vi "Cal BC (Numeric).vi"(8 "error in (no error)":errorcluster, 10 "BC in":variant, 11 "Domain_Steady_2D_Rect in":refnum<class "NI_Domain_Steady_2D_Rect.lvclass">) -> (0 "error out":errorcluster, 2 "BC out":variant, 3 "Domain_Steady_2D_Rect out":refnum<class "NI_Domain_Steady_2D_Rect.lvclass">)   [LabVIEW 2017, in "NI_PDE.lvlib" / "NI_Domain_Steady_2D_Rect.lvclass"]
uses:
  <vilib>/gmath/pde.llb/DomainClass/Domain_Steady_2D_Rect/NI_Domain_Steady_2D_Rect.lvclass
  <vilib>/gmath/pde.llb/BCClass/BC_Steady_2D_Numeric/BC Data.ctl
  <vilib>/gmath/pde.llb/Common/PDE_BC Type.ctl
  <vilib>/gmath/pde.llb/Common/PDE_BC Position 2D.ctl
  <vilib>/gmath/pde.llb/DomainClass/Domain_Steady_2D_Rect/NI_Domain_Steady_2D_Rect.lvclass/NI_Domain_Steady_2D_Rect.ctl
  <vilib>/gmath/NI_PDE.lvlib
  <vilib>/gmath/pde.llb/BCClass/BC_Steady_2D_Numeric/NI_BC_Steady_2D_Numeric.lvclass
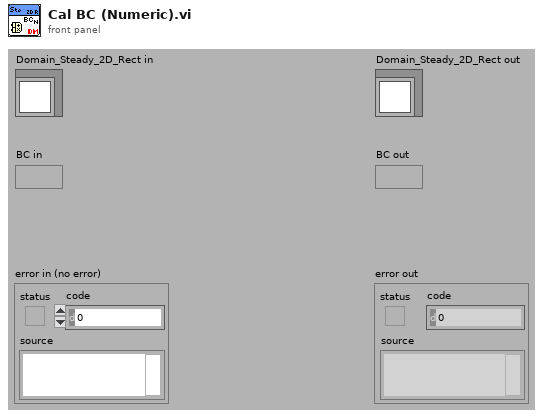
[diagram p1: front panel]
types:
  T1 = typedef "NI_PDE.lvlib/NI_BC_Steady_2D_Numeric.lvclass/BC Data.ctl" = cluster{"type":T2, "position":T3, "G":dbl[]}
  T2 = typedef "NI_PDE.lvlib/PDE_BC Type.ctl" = i32
  T3 = typedef "NI_PDE.lvlib/PDE_BC Position 2D.ctl" = i32
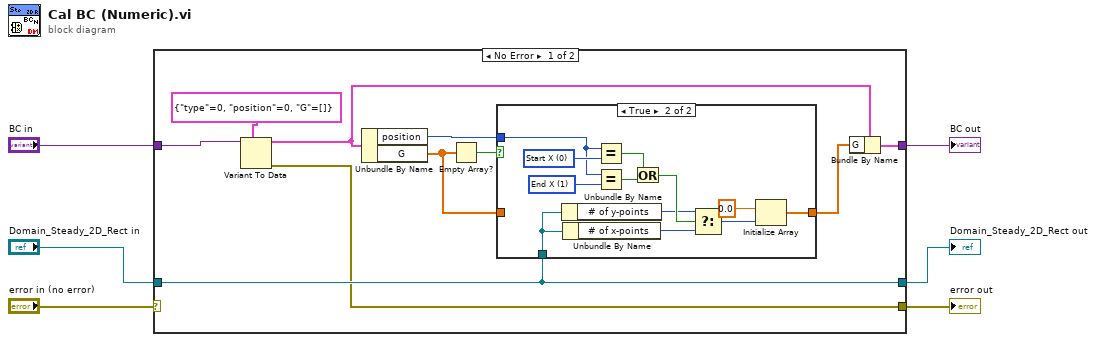
[diagram p0: block diagram]
diagram:
  n1 = case shown="No Error" "error in (no error)" {
    selector: "error in (no error)" -> [_ w32]
    tunnel: "Domain_Steady_2D_Rect in" -> [w8 w31]
    tunnel: [w8 w31] -> w6
    tunnel: [w7 w32] -> w5
    tunnel: [w9 w30] -> w2
    tunnel: "BC in" -> [w13 w30]
    frame No Error {
      n2 = Variant To Data(type=T1 {"type"=0, "position"=0, "G"=[]} ("BC data"), Variant=w13) -> (data=w11:T1, error out=w7:errorcluster)  [unwired: 1 in]
      n3 = Unbundle By Name(w11) -> ("position"=w12:T3, "G"=w15:dbl[])
      n4 = Empty Array?(array=w15) -> (empty?=w16:bool)
      n5 = case shown="True" w16 {
        tunnel: w15 -> [w17 _]
        tunnel: [w17 w29] -> w10
        tunnel: w12 -> [_ w19]
        tunnel: w8 -> [_ w18]
        frame False {
        }
        frame True {
          w26 = T3 1 items=["Start X", "End X", "Start Y", "End Y"] ("y")
          w27 = T3 0 items=["Start X", "End X", "Start Y", "End Y"] ("y")
          n6 = Unbundle By Name(w18) -> ("# of y-points"=w22:i32)
          n7 = Unbundle By Name(w18) -> ("# of x-points"=w20:i32)
          n8 = Equal?(x=w19, y=w27) -> (x = y?=w25:bool)
          n9 = Equal?(x=w19, y=w26) -> (x = y?=w24:bool)
          n10 = Or(x=w25, y=w24) -> (x .or. y?=w23:bool)
          n11 = Select(t=w22, s=w23, f=w20) -> (s? t:f=w21:i32)
          n12 = Initialize Array(0.0 ("element"), w21) -> (w29:dbl[])
        }
      }
      n13 = Bundle By Name(cluster=w11, "G"=w10) -> (w9:T1)
    }
    frame Error {
    }
  }
  "Domain_Steady_2D_Rect out" <- w6
  "error out" <- w5
  "BC out" <- w2
